vi "Test Magnet.vi"(8 "error in (no error)":errorcluster) -> (0 "error out":errorcluster)   [LabVIEW 2019]
uses:
  lvsrc/Instrument Types/Cryostat/Instrument.Cryostat.lvclass
  <vilib>/addons/_JKI Toolkits/Caraya/classes/Assert/Assert Error.vi
  <vilib>/addons/_JKI Toolkits/Caraya/classes/Assert/Assert Almost Equal_Float.vi
  <vilib>/addons/_JKI Toolkits/Caraya/classes/Test/Test.lvclass
  <vilib>/addons/_JKI Toolkits/Caraya/classes/Assert/Assert.lvclass
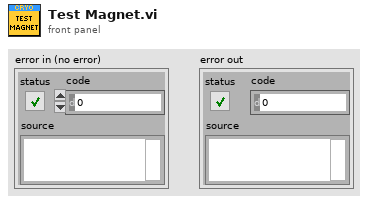
[diagram p1: front panel]
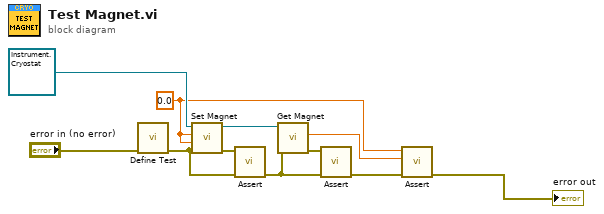
[diagram p0: block diagram]
diagram:
  w2 = 0.0 ("Angle (°)")
  n1 = call <vilib>:"Define Test.vi"("error in (no error)"="error in (no error)") -> ("error out"=w1:errorcluster)  [unwired: 10 in]
  n2 = call-dynamic "Set Magnet.vi"("error in (no error)"=w1, "Target Rate (T/min)"=w2, "Target Field (T)"=w2, "Instrument.Cryostat in"=refnum<class "Instrument.Cryostat.lvclass"> refnum) -> ("error out"=w9:errorcluster, "Instrument.Cryostat out"=w7:refnum<class "Instrument.Cryostat.lvclass">)  [unwired: 6 in]
  n3 = call-poly <vilib>:"Assert.vi"("error in (no error)"=w1, "Error?"=w9) -> ("error out"=w5:errorcluster)  [unwired: 9 in]
  n4 = call-dynamic "Get Magnet.vi"("error in (no error)"=w5, "Instrument.Cryostat in"=w7) -> ("error out"=w10:errorcluster, "B Field (T)"=w3:dbl)  [unwired: 5 in, 3 out]
  n5 = call-poly <vilib>:"Assert.vi"("error in (no error)"=w5, "Error?"=w10) -> ("error out"=w11:errorcluster)  [unwired: 9 in]
  n6 = call-poly <vilib>:"Assert.vi"("error in (no error)"=w11, "Y"=w3, "X"=w2) -> ("error out"=→"error out":errorcluster)  [unwired: 8 in]
